vi "CRYGet All Except Common Between Two Arrays.vi"(9 "B":dbl[](array[numeric]), 11 "A":dbl[](array[numeric])) -> (3 "Result":dbl[](array[numeric]))   [LabVIEW 2013]
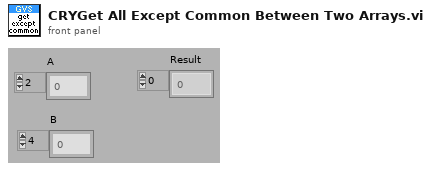
[diagram p1: front panel]
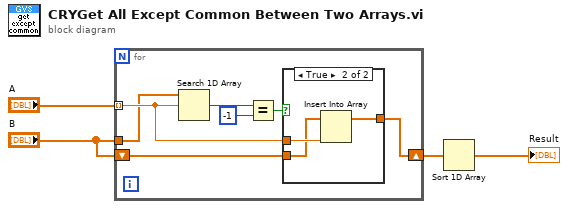
[diagram p0: block diagram]
diagram:
  n1 = for {
    tunnel: "A" -> [w8] mode=indexing
    shift-right: [w5] -> w2
    shift-left: "B" -> [w6]
    tunnel: "B" -> [w7]
    n2 = Search 1D Array(1D array=w7, element=w8) -> (index of element=w11:i32)  [unwired: 1 out]
    n3 = Equal?(x=w11, y=-1) -> (x = y?=w9:bool)
    n4 = case shown="True" w9 {
      tunnel: w8 -> [_ w15]
      tunnel: w6 -> [w12 w14]
      tunnel: [w12 w13] -> w5
      frame False {
      }
      frame True {
        n5 = Insert Into Array(array=w14, new element=w15) -> (w13:dbl[])  [unwired: 1 in]
      }
    }
  }
  n6 = Sort 1D Array(array=w2) -> (sorted array=→"Result":dbl[])
